vi "WheelEncoderCountToDistance.vi"(1 "EncoderCounts":i32, 2 "CountsPerRevolution":i32=4096, 3 "WheelDiameter(in)":dbl=4.0) -> (0 "Output(in)":dbl)   [LabVIEW 2017]
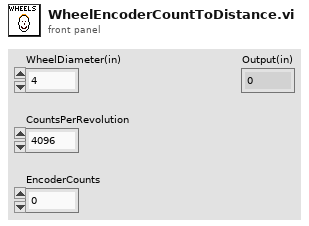
[diagram p1: front panel]
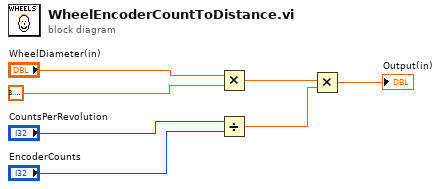
[diagram p0: block diagram]
diagram:
  n1 = Multiply(x="WheelDiameter(in)", y=3.141592653589793) -> (x*y=w5:dbl)
  n2 = Divide(x="CountsPerRevolution", y="EncoderCounts") -> (x/y=w3:dbl)
  n3 = Multiply(x=w5, y=w3) -> (x*y=→"Output(in)":dbl)
